vi "Lab Panel V4.86.vi"() -> ()   [LabVIEW 2013] (continued)
                n1197 = case shown="True" w2168 {
                  tunnel: w2173 -> [_ w2177]
                  tunnel: w2167 -> [_ w2180]
                  frame False {
                  }
                  frame True {
                    n1198 = local read "SET LAB01-1"() -> (w2179:T5)
                    n1199 = local read "TDMS LAB01-1"() -> (w2176:refnum<k34>)
                    n1200 = Unbundle(w2177) -> ("CYCLE"=w2181:dbl)  [unwired: 2 out]
                    n1201 = Unbundle(w2179) -> ("T-RISE mins"=w2178:dbl)  [unwired: 4 out]
                    n1202 = Greater Or Equal?(x=w2181, y=w2180) -> (x >= y?=w2182:bool)
                    n1203 = case shown="True" w2182 {
                      tunnel: w2178 -> [w2185 _]
                      tunnel: w2177 -> [w2184 _]
                      tunnel: w2176 -> [w2183 _]
                      frame True {
                        n1204 = stacked-sequence {
                          tunnel: w2185 -> [w2188 _]
                          tunnel: w2184 -> [_ w2193]
                          tunnel: w2183 -> [w2186 _]
                          frame #0 {
                            n1205 = Build Array("T-RISE") -> (w2190:string[])
                            n1206 = Build Array(w2188) -> (w2189:dbl[])
                            n1207 = TDMS Write(0:w2186, 5:"TEST PASS", 7:w2190, 9:w2189) -> (15:w2192:errorcluster)  [unwired: 2 in, 3 out]
                            n1208 = local write "data file error"(w2192) -> ()
                          }
                          frame #1 {
                            n1209 = Bundle(cluster=w2193, "STATUS"="T-RISE PASS") -> (w2195:T4)  [unwired: 2 in]
                            n1210 = local write "RESULT LAB01-1"(TRUE) -> ()
                            n1211 = local write "DISP LAB01-1"(w2195) -> ()
                          }
                        }
                      }
                      frame False {
                      }
                    }
                  }
                }
              }
              frame #1 {
                # "LAB01-2"
                n1212 = Equal?(x=w2198, y=2) -> (x = y?=w2201:bool)
                n1213 = local read "DISP LAB01-2"() -> (w2203:T4)
                n1214 = Unbundle(w2203) -> ("STATUS"=w2204:string)  [unwired: 2 out]
                n1215 = Equal?(x=w2204, y="RUN") -> (x = y?=w2200:bool)
                n1216 = And(x=w2200, y=w2201) -> (x .and. y?=w2199:bool)
                n1217 = case shown="True" w2199 {
                  tunnel: w2203 -> [_ w2207]
                  tunnel: w2197 -> [_ w2210]
                  frame False {
                  }
                  frame True {
                    n1218 = local read "SET LAB01-2"() -> (w2209:T5)
                    n1219 = local read "TDMS LAB01-2"() -> (w2206:refnum<k34>)
                    n1220 = Unbundle(w2207) -> ("CYCLE"=w2211:dbl)  [unwired: 2 out]
                    n1221 = Unbundle(w2209) -> ("T-RISE mins"=w2208:dbl)  [unwired: 4 out]
                    n1222 = Greater Or Equal?(x=w2211, y=w2210) -> (x >= y?=w2212:bool)
                    n1223 = case shown="True" w2212 {
                      tunnel: w2208 -> [w2215 _]
                      tunnel: w2207 -> [w2214 _]
                      tunnel: w2206 -> [w2213 _]
                      frame True {
                        n1224 = stacked-sequence {
                          tunnel: w2215 -> [w2218 _]
                          tunnel: w2214 -> [_ w2223]
                          tunnel: w2213 -> [w2216 _]
                          frame #0 {
                            n1225 = Build Array("T-RISE") -> (w2220:string[])
                            n1226 = Build Array(w2218) -> (w2219:dbl[])
                            n1227 = TDMS Write(0:w2216, 5:"TEST PASS", 7:w2220, 9:w2219) -> (15:w2222:errorcluster)  [unwired: 2 in, 3 out]
                            n1228 = local write "data file error"(w2222) -> ()
                          }
                          frame #1 {
                            n1229 = Bundle(cluster=w2223, "STATUS"="T-RISE PASS") -> (w2225:T4)  [unwired: 2 in]
                            n1230 = local write "RESULT LAB01-2"(TRUE) -> ()
                            n1231 = local write "DISP LAB01-2"(w2225) -> ()
                          }
                        }
                      }
                      frame False {
                      }
                    }
                  }
                }
              }
              frame #2 {
                # "LAB02-1"
                n1232 = Equal?(x=w2228, y=2) -> (x = y?=w2231:bool)
                n1233 = local read "DISP LAB02-1"() -> (w2233:T4)
                n1234 = Unbundle(w2233) -> ("STATUS"=w2234:string)  [unwired: 2 out]
                n1235 = Equal?(x=w2234, y="RUN") -> (x = y?=w2230:bool)
                n1236 = And(x=w2230, y=w2231) -> (x .and. y?=w2229:bool)
                n1237 = case shown="True" w2229 {
                  tunnel: w2233 -> [_ w2237]
                  tunnel: w2227 -> [_ w2240]
                  frame False {
                  }
                  frame True {
                    n1238 = local read "SET LAB02-1"() -> (w2239:T5)
                    n1239 = local read "TDMS LAB02-1"() -> (w2236:refnum<k34>)
                    n1240 = Unbundle(w2237) -> ("CYCLE"=w2241:dbl)  [unwired: 2 out]
                    n1241 = Unbundle(w2239) -> ("T-RISE mins"=w2238:dbl)  [unwired: 4 out]
                    n1242 = Greater Or Equal?(x=w2241, y=w2240) -> (x >= y?=w2242:bool)
                    n1243 = case shown="True" w2242 {
                      tunnel: w2238 -> [w2245 _]
                      tunnel: w2237 -> [w2244 _]
                      tunnel: w2236 -> [w2243 _]
                      frame True {
                        n1244 = stacked-sequence {
                          tunnel: w2245 -> [w2248 _]
                          tunnel: w2244 -> [_ w2253]
                          tunnel: w2243 -> [w2246 _]
                          frame #0 {
                            n1245 = Build Array("T-RISE") -> (w2250:string[])
                            n1246 = Build Array(w2248) -> (w2249:dbl[])
                            n1247 = TDMS Write(0:w2246, 5:"TEST PASS", 7:w2250, 9:w2249) -> (15:w2252:errorcluster)  [unwired: 2 in, 3 out]
                            n1248 = local write "data file error"(w2252) -> ()
                          }
                          frame #1 {
                            n1249 = Bundle(cluster=w2253, "STATUS"="T-RISE PASS") -> (w2255:T4)  [unwired: 2 in]
                            n1250 = local write "RESULT LAB02-1"(TRUE) -> ()
                            n1251 = local write "DISP LAB02-1"(w2255) -> ()
                          }
                        }
                      }
                      frame False {
                      }
                    }
                  }
                }
              }
              frame #3 {
                # "LAB02-2"
                n1252 = Equal?(x=w2258, y=2) -> (x = y?=w2261:bool)
                n1253 = local read "DISP LAB02-2"() -> (w2263:T4)
                n1254 = Unbundle(w2263) -> ("STATUS"=w2264:string)  [unwired: 2 out]
                n1255 = Equal?(x=w2264, y="RUN") -> (x = y?=w2260:bool)
                n1256 = And(x=w2260, y=w2261) -> (x .and. y?=w2259:bool)
                n1257 = case shown="True" w2259 {
                  tunnel: w2263 -> [_ w2267]
                  tunnel: w2257 -> [_ w2270]
                  frame False {
                  }
                  frame True {
                    n1258 = local read "SET LAB02-2"() -> (w2269:T5)
                    n1259 = local read "TDMS LAB02-2"() -> (w2266:refnum<k34>)
                    n1260 = Unbundle(w2267) -> ("CYCLE"=w2271:dbl)  [unwired: 2 out]
                    n1261 = Unbundle(w2269) -> ("T-RISE mins"=w2268:dbl)  [unwired: 4 out]
                    n1262 = Greater Or Equal?(x=w2271, y=w2270) -> (x >= y?=w2272:bool)
                    n1263 = case shown="True" w2272 {
                      tunnel: w2268 -> [w2275 _]
                      tunnel: w2267 -> [w2274 _]
                      tunnel: w2266 -> [w2273 _]
                      frame True {
                        n1264 = stacked-sequence {
                          tunnel: w2275 -> [w2278 _]
                          tunnel: w2274 -> [_ w2283]
                          tunnel: w2273 -> [w2276 _]
                          frame #0 {
                            n1265 = Build Array("T-RISE") -> (w2280:string[])
                            n1266 = Build Array(w2278) -> (w2279:dbl[])
                            n1267 = TDMS Write(0:w2276, 5:"TEST PASS", 7:w2280, 9:w2279) -> (15:w2282:errorcluster)  [unwired: 2 in, 3 out]
                            n1268 = local write "data file error"(w2282) -> ()
                          }
                          frame #1 {
                            n1269 = Bundle(cluster=w2283, "STATUS"="T-RISE PASS") -> (w2285:T4)  [unwired: 2 in]
                            n1270 = local write "RESULT LAB02-2"(TRUE) -> ()
                            n1271 = local write "DISP LAB02-2"(w2285) -> ()
                          }
                        }
                      }
                      frame False {
                      }
                    }
                  }
                }
              }
              frame #4 {
                # "LAB03-1"
                n1272 = Equal?(x=w2288, y=2) -> (x = y?=w2291:bool)
                n1273 = local read "DISP LAB03-1"() -> (w2293:T4)
                n1274 = Unbundle(w2293) -> ("STATUS"=w2294:string)  [unwired: 2 out]
                n1275 = Equal?(x=w2294, y="RUN") -> (x = y?=w2290:bool)
                n1276 = And(x=w2290, y=w2291) -> (x .and. y?=w2289:bool)
                n1277 = case shown="True" w2289 {
                  tunnel: w2293 -> [_ w2297]
                  tunnel: w2287 -> [_ w2300]
                  frame False {
                  }
                  frame True {
                    n1278 = local read "SET LAB03-1"() -> (w2299:T5)
                    n1279 = local read "TDMS LAB03-1"() -> (w2296:refnum<k34>)
                    n1280 = Unbundle(w2297) -> ("CYCLE"=w2301:dbl)  [unwired: 2 out]
                    n1281 = Unbundle(w2299) -> ("T-RISE mins"=w2298:dbl)  [unwired: 4 out]
                    n1282 = Greater Or Equal?(x=w2301, y=w2300) -> (x >= y?=w2302:bool)
                    n1283 = case shown="True" w2302 {
                      tunnel: w2298 -> [w2305 _]
                      tunnel: w2297 -> [w2304 _]
                      tunnel: w2296 -> [w2303 _]
                      frame True {
                        n1284 = stacked-sequence {
                          tunnel: w2305 -> [w2308 _]
                          tunnel: w2304 -> [_ w2313]
                          tunnel: w2303 -> [w2306 _]
                          frame #0 {
                            n1285 = Build Array("T-RISE") -> (w2310:string[])
                            n1286 = Build Array(w2308) -> (w2309:dbl[])
                            n1287 = TDMS Write(0:w2306, 5:"TEST PASS", 7:w2310, 9:w2309) -> (15:w2312:errorcluster)  [unwired: 2 in, 3 out]
                            n1288 = local write "data file error"(w2312) -> ()
                          }
                          frame #1 {
                            n1289 = Bundle(cluster=w2313, "STATUS"="T-RISE PASS") -> (w2315:T4)  [unwired: 2 in]
                            n1290 = local write "RESULT LAB03-1"(TRUE) -> ()
                            n1291 = local write "DISP LAB03-1"(w2315) -> ()
                          }
                        }
                      }
                      frame False {
                      }
                    }
                  }
                }
              }
              frame #5 {
                # "LAB03-2"
                n1292 = Equal?(x=w2318, y=2) -> (x = y?=w2321:bool)
                n1293 = local read "DISP LAB03-2"() -> (w2323:T4)
                n1294 = Unbundle(w2323) -> ("STATUS"=w2324:string)  [unwired: 2 out]
                n1295 = Equal?(x=w2324, y="RUN") -> (x = y?=w2320:bool)
                n1296 = And(x=w2320, y=w2321) -> (x .and. y?=w2319:bool)
                n1297 = case shown="True" w2319 {
                  tunnel: w2323 -> [_ w2327]
                  tunnel: w2317 -> [_ w2330]
                  frame False {
                  }
                  frame True {
                    n1298 = local read "SET LAB03-2"() -> (w2329:T5)
                    n1299 = local read "TDMS LAB03-2"() -> (w2326:refnum<k34>)
                    n1300 = Unbundle(w2327) -> ("CYCLE"=w2331:dbl)  [unwired: 2 out]
                    n1301 = Unbundle(w2329) -> ("T-RISE mins"=w2328:dbl)  [unwired: 4 out]
                    n1302 = Greater Or Equal?(x=w2331, y=w2330) -> (x >= y?=w2332:bool)
                    n1303 = case shown="True" w2332 {
                      tunnel: w2328 -> [w2335 _]
                      tunnel: w2327 -> [w2334 _]
                      tunnel: w2326 -> [w2333 _]
                      frame True {
                        n1304 = stacked-sequence {
                          tunnel: w2335 -> [w2338 _]
                          tunnel: w2334 -> [_ w2343]
                          tunnel: w2333 -> [w2336 _]
                          frame #0 {
                            n1305 = Build Array("T-RISE") -> (w2340:string[])
                            n1306 = Build Array(w2338) -> (w2339:dbl[])
                            n1307 = TDMS Write(0:w2336, 5:"TEST PASS", 7:w2340, 9:w2339) -> (15:w2342:errorcluster)  [unwired: 2 in, 3 out]
                            n1308 = local write "data file error"(w2342) -> ()
                          }
                          frame #1 {
                            n1309 = Bundle(cluster=w2343, "STATUS"="T-RISE PASS") -> (w2345:T4)  [unwired: 2 in]
                            n1310 = local write "RESULT LAB03-2"(TRUE) -> ()
                            n1311 = local write "DISP LAB03-2"(w2345) -> ()
                          }
                        }
                      }
                      frame False {
                      }
                    }
                  }
                }
              }
              frame #6 {
                # "LAB04-1"
                n1312 = Equal?(x=w2348, y=2) -> (x = y?=w2351:bool)
                n1313 = local read "DISP LAB04-1"() -> (w2353:T4)
                n1314 = Unbundle(w2353) -> ("STATUS"=w2354:string)  [unwired: 2 out]
                n1315 = Equal?(x=w2354, y="RUN") -> (x = y?=w2350:bool)
                n1316 = And(x=w2350, y=w2351) -> (x .and. y?=w2349:bool)
                n1317 = case shown="True" w2349 {
                  tunnel: w2353 -> [_ w2357]
                  tunnel: w2347 -> [_ w2360]
                  frame False {
                  }
                  frame True {
                    n1318 = local read "SET LAB04-1"() -> (w2359:T5)
                    n1319 = local read "TDMS LAB04-1"() -> (w2356:refnum<k34>)
                    n1320 = Unbundle(w2357) -> ("CYCLE"=w2361:dbl)  [unwired: 2 out]
                    n1321 = Unbundle(w2359) -> ("T-RISE mins"=w2358:dbl)  [unwired: 4 out]
                    n1322 = Greater Or Equal?(x=w2361, y=w2360) -> (x >= y?=w2362:bool)
                    n1323 = case shown="True" w2362 {
                      tunnel: w2358 -> [w2365 _]
                      tunnel: w2357 -> [w2364 _]
                      tunnel: w2356 -> [w2363 _]
                      frame True {
                        n1324 = stacked-sequence {
                          tunnel: w2365 -> [w2368 _]
                          tunnel: w2364 -> [_ w2373]
                          tunnel: w2363 -> [w2366 _]
                          frame #0 {
                            n1325 = Build Array("T-RISE") -> (w2370:string[])
                            n1326 = Build Array(w2368) -> (w2369:dbl[])
                            n1327 = TDMS Write(0:w2366, 5:"TEST PASS", 7:w2370, 9:w2369) -> (15:w2372:errorcluster)  [unwired: 2 in, 3 out]
                            n1328 = local write "data file error"(w2372) -> ()
                          }
                          frame #1 {
                            n1329 = Bundle(cluster=w2373, "STATUS"="T-RISE PASS") -> (w2375:T4)  [unwired: 2 in]
                            n1330 = local write "RESULT LAB04-1"(TRUE) -> ()
                            n1331 = local write "DISP LAB04-1"(w2375) -> ()
                          }
                        }
                      }
                      frame False {
                      }
                    }
                  }
                }
              }
              frame #7 {
                # "LAB04-2"
                n1332 = Equal?(x=w2378, y=2) -> (x = y?=w2381:bool)
                n1333 = local read "DISP LAB04-2"() -> (w2383:T4)
                n1334 = Unbundle(w2383) -> ("STATUS"=w2384:string)  [unwired: 2 out]
                n1335 = Equal?(x=w2384, y="RUN") -> (x = y?=w2380:bool)
                n1336 = And(x=w2380, y=w2381) -> (x .and. y?=w2379:bool)
                n1337 = case shown="True" w2379 {
                  tunnel: w2383 -> [_ w2387]
                  tunnel: w2377 -> [_ w2390]
                  frame False {
                  }
                  frame True {
                    n1338 = local read "SET LAB04-2"() -> (w2389:T5)
                    n1339 = local read "TDMS LAB04-2"() -> (w2386:refnum<k34>)
                    n1340 = Unbundle(w2387) -> ("CYCLE"=w2391:dbl)  [unwired: 2 out]
                    n1341 = Unbundle(w2389) -> ("T-RISE mins"=w2388:dbl)  [unwired: 4 out]
                    n1342 = Greater Or Equal?(x=w2391, y=w2390) -> (x >= y?=w2392:bool)
                    n1343 = case shown="True" w2392 {
                      tunnel: w2388 -> [w2395 _]
                      tunnel: w2387 -> [w2394 _]
                      tunnel: w2386 -> [w2393 _]
                      frame True {
                        n1344 = stacked-sequence {
                          tunnel: w2395 -> [w2398 _]
                          tunnel: w2394 -> [_ w2403]
                          tunnel: w2393 -> [w2396 _]
                          frame #0 {
                            n1345 = Build Array("T-RISE") -> (w2400:string[])
                            n1346 = Build Array(w2398) -> (w2399:dbl[])
                            n1347 = TDMS Write(0:w2396, 5:"TEST PASS", 7:w2400, 9:w2399) -> (15:w2402:errorcluster)  [unwired: 2 in, 3 out]
                            n1348 = local write "data file error"(w2402) -> ()
                          }
                          frame #1 {
                            n1349 = Bundle(cluster=w2403, "STATUS"="T-RISE PASS") -> (w2405:T4)  [unwired: 2 in]
                            n1350 = local write "RESULT LAB04-2"(TRUE) -> ()
                            n1351 = local write "DISP LAB04-2"(w2405) -> ()
                          }
                        }
                      }
                      frame False {
                      }
                    }
                  }
                }
              }
              frame #8 {
                # "LAB05-1"
                n1352 = Equal?(x=w2408, y=2) -> (x = y?=w2411:bool)
                n1353 = local read "DISP LAB05-1"() -> (w2413:T4)
                n1354 = Unbundle(w2413) -> ("STATUS"=w2414:string)  [unwired: 2 out]
                n1355 = Equal?(x=w2414, y="RUN") -> (x = y?=w2410:bool)
                n1356 = And(x=w2410, y=w2411) -> (x .and. y?=w2409:bool)
                n1357 = case shown="True" w2409 {
                  tunnel: w2413 -> [_ w2417]
                  tunnel: w2407 -> [_ w2420]
                  frame False {
                  }
                  frame True {
                    n1358 = local read "SET LAB05-1"() -> (w2419:T5)
                    n1359 = local read "TDMS LAB05-1"() -> (w2416:refnum<k34>)
                    n1360 = Unbundle(w2417) -> ("CYCLE"=w2421:dbl)  [unwired: 2 out]
                    n1361 = Unbundle(w2419) -> ("T-RISE mins"=w2418:dbl)  [unwired: 4 out]
                    n1362 = Greater Or Equal?(x=w2421, y=w2420) -> (x >= y?=w2422:bool)
                    n1363 = case shown="True" w2422 {
                      tunnel: w2418 -> [w2425 _]
                      tunnel: w2417 -> [w2424 _]
                      tunnel: w2416 -> [w2423 _]
                      frame True {
                        n1364 = stacked-sequence {
                          tunnel: w2425 -> [w2428 _]
                          tunnel: w2424 -> [_ w2433]
                          tunnel: w2423 -> [w2426 _]
                          frame #0 {
                            n1365 = Build Array("T-RISE") -> (w2430:string[])
                            n1366 = Build Array(w2428) -> (w2429:dbl[])
                            n1367 = TDMS Write(0:w2426, 5:"TEST PASS", 7:w2430, 9:w2429) -> (15:w2432:errorcluster)  [unwired: 2 in, 3 out]
                            n1368 = local write "data file error"(w2432) -> ()
                          }
                          frame #1 {
                            n1369 = Bundle(cluster=w2433, "STATUS"="T-RISE PASS") -> (w2435:T4)  [unwired: 2 in]
                            n1370 = local write "RESULT LAB05-1"(TRUE) -> ()
                            n1371 = local write "DISP LAB05-1"(w2435) -> ()
                          }
                        }
                      }
                      frame False {
                      }
                    }
                  }
                }
              }
              frame #9 {
                # "LAB05-2"
                n1372 = Equal?(x=w2438, y=2) -> (x = y?=w2441:bool)
                n1373 = local read "DISP LAB05-2"() -> (w2443:T4)
                n1374 = Unbundle(w2443) -> ("STATUS"=w2444:string)  [unwired: 2 out]
                n1375 = Equal?(x=w2444, y="RUN") -> (x = y?=w2440:bool)
                n1376 = And(x=w2440, y=w2441) -> (x .and. y?=w2439:bool)
                n1377 = case shown="True" w2439 {
                  tunnel: w2443 -> [_ w2447]
                  tunnel: w2437 -> [_ w2450]
                  frame False {
                  }
                  frame True {
                    n1378 = local read "SET LAB05-2"() -> (w2449:T5)
                    n1379 = local read "TDMS LAB05-2"() -> (w2446:refnum<k34>)
                    n1380 = Unbundle(w2447) -> ("CYCLE"=w2451:dbl)  [unwired: 2 out]
                    n1381 = Unbundle(w2449) -> ("T-RISE mins"=w2448:dbl)  [unwired: 4 out]
                    n1382 = Greater Or Equal?(x=w2451, y=w2450) -> (x >= y?=w2452:bool)
                    n1383 = case shown="True" w2452 {
                      tunnel: w2448 -> [w2455 _]
                      tunnel: w2447 -> [w2454 _]
                      tunnel: w2446 -> [w2453 _]
                      frame True {
                        n1384 = stacked-sequence {
                          tunnel: w2455 -> [w2458 _]
                          tunnel: w2454 -> [_ w2463]
                          tunnel: w2453 -> [w2456 _]
                          frame #0 {
                            n1385 = Build Array("T-RISE") -> (w2460:string[])
                            n1386 = Build Array(w2458) -> (w2459:dbl[])
                            n1387 = TDMS Write(0:w2456, 5:"TEST PASS", 7:w2460, 9:w2459) -> (15:w2462:errorcluster)  [unwired: 2 in, 3 out]
                            n1388 = local write "data file error"(w2462) -> ()
                          }
                          frame #1 {
                            n1389 = Bundle(cluster=w2463, "STATUS"="T-RISE PASS") -> (w2465:T4)  [unwired: 2 in]
                            n1390 = local write "RESULT LAB05-2"(TRUE) -> ()
                            n1391 = local write "DISP LAB05-2"(w2465) -> ()
                          }
                        }
                      }
                      frame False {
                      }
                    }
                  }
                }
              }
            }
          }
          frame #6 {
            # "end test & close test files"
            n1392 = local read "MAIL SETTINGS"() -> (w2471:T6)
            n1393 = Unbundle(w2471) -> ("OUT SERVER ADDRESS"=w2470:string, "FROM ACCOUNT"=w2469:string)  [unwired: 5 out]
            n1394 = stacked-sequence {
              tunnel: w2481 -> [_ _ _ _ _ _ _ _ _ _]
              tunnel: w2482 -> [_ _ _ _ _ _ _ _ _ _]
              tunnel: w2480 -> [_ _ _ _ _ _ _ _ _ _]
              tunnel: w2479 -> [_ _ _ _ _ _ _ _ _ _]
              tunnel: w2478 -> [_ _ _ _ _ _ _ _ _ _]
              tunnel: w2477 -> [_ _ _ _ _ _ _ _ _ _]
              tunnel: w2476 -> [_ _ _ _ _ _ _ _ _ _]
              tunnel: w2475 -> [_ _ _ _ _ _ _ _ _ _]
              tunnel: w2474 -> [_ _ _ _ _ _ _ _ _ _]
              tunnel: w2473 -> [_ _ _ _ _ _ _ _ _ _]
              tunnel: w2470 -> [w2486 w2538 w2586 w2633 w2680 w2727 w2774 w2821 w2868 w2915]
              tunnel: w2469 -> [w2485 w2537 w2585 w2632 w2679 w2726 w2773 w2820 w2867 w2914]
              tunnel: "Mail Test File To:" -> [w2484 w2536 w2584 w2631 w2678 w2725 w2772 w2819 w2866 w2913]
              tunnel: "Mail Test Fail" -> [w2483 w2535 w2583 w2630 w2677 w2724 w2771 w2818 w2865 w2912]
              frame #0 {
                # "LAB01-1"
                n1395 = local read "DISP LAB01-1"() -> (w2490:T4)
                n1396 = local read "run lab01-1"() -> (w2487:bool)
                n1397 = local read "TDMS LAB01-1"() -> (w2488:refnum<k34>)
                n1398 = Unbundle(w2490) -> ("CYCLE"=w2491:dbl, "STATUS"=w2489:string)  [unwired: 1 out]
                n1399 = case shown="True" w2487 {
                  tunnel: w2491 -> [_ w2497]
                  tunnel: w2490 -> [_ w2499]
                  tunnel: w2489 -> [_ w2496]
                  tunnel: w2488 -> [_ w2498]
                  tunnel: w2486 -> [_ w2495]
                  tunnel: w2485 -> [_ w2494]
                  tunnel: w2484 -> [_ w2493]
                  tunnel: w2483 -> [_ w2492]
                  frame False {
                  }
                  frame True {
                    n1400 = Not Equal?(x=w2496, y="RUN") -> (x != y?=w2500:bool)
                    n1401 = Greater?(x=w2497, y=2.0) -> (0:w2502:bool)
                    n1402 = And(x=w2502, y=w2500) -> (x .and. y?=w2501:bool)
                    n1403 = case shown="True" w2501 {
                      tunnel: w2499 -> [_ w2512]
                      tunnel: w2498 -> [_ w2511]
                      tunnel: w2497 -> [_ w2510]
                      tunnel: w2496 -> [_ w2509]
                      tunnel: w2495 -> [_ w2508]
                      tunnel: w2494 -> [_ w2507]
                      tunnel: w2493 -> [_ w2506]
                      tunnel: w2492 -> [_ w2505]
                      frame False {
                      }
                      frame True {
                        n1404 = stacked-sequence {
                          tunnel: w2512 -> [w2516 _ _]
                          tunnel: w2511 -> [_ w2518 _]
                          tunnel: w2510 -> [_ _ _]
                          tunnel: w2509 -> [_ _ w2524]
                          tunnel: w2508 -> [_ _ w2523]
                          tunnel: w2507 -> [_ _ w2522]
                          tunnel: w2506 -> [_ _ w2521]
                          tunnel: w2505 -> [_ _ w2520]
                          frame #0 {
                            w2513 = FALSE
                            n1405 = local write "mail control"("END") -> ()
                            n1406 = Bundle(cluster=w2516) -> (w2515:T4)  [unwired: 3 in]
                            n1407 = local write "DISP LAB01-1"(w2515) -> ()
                            n1408 = local write "O/I  LAB01-1"(w2513) -> ()
                            n1409 = local write "run lab01-1"(w2513) -> ()
                            n1410 = local write "RUN LAB01-1"(w2513) -> ()
                          }
                          frame #1 {
                            n1411 = TDMS Close(11:w2518) -> (0:w2517:errorcluster)  [unwired: 1 in, 1 out]
                            n1412 = local write "data file error"(w2517) -> ()
                          }
                          frame #2 {
                            n1413 = stacked-sequence {
                              tunnel: "LAB01-1" -> [w2526 w2528 _]
                              tunnel: w2524 -> [_ w2534 _]
                              tunnel: w2523 -> [_ w2533 _]
                              tunnel: w2522 -> [_ w2532 _]
                              tunnel: w2521 -> [_ w2531 _]
                              tunnel: w2520 -> [_ w2530 _]
                              frame #0 {
                                n1414 = call "sub vi - defrag tdms v1.vi"("panel id"=w2526) -> ("error out"=w2525:errorcluster)  [unwired: 10 in]
                                n1415 = local write "data file error"(w2525) -> ()
                              }
                              frame #1 {
                                n1416 = Bundle("STATUS"=w2534, "OUT SERVER ADDRESS"=w2533, "FROM ACCOUNT"=w2532, "Mail Test File To:"=w2531, "Mail Test Fail"=w2530) -> (w2527:T23)  [unwired: 1 in]
                                n1417 = call "Save data file to network drive v3.vi"("Input Cluster"=w2527, "panel id"=w2528) -> ("network file save error"=w2529:errorcluster)  [unwired: 8 in, 1 out]
                                n1418 = local write "data file error"(w2529) -> ()
                              }
                              frame #2 {
                              }
                            }
                          }
                        }
                      }
                    }
                  }
                }
              }
              frame #1 {
                # "LAB01-2"
                n1419 = local read "run lab01-2"() -> (w2539:bool)
                n1420 = case shown="True" w2539 {
                  tunnel: w2538 -> [_ w2543]
                  tunnel: w2537 -> [_ w2542]
                  tunnel: w2536 -> [_ w2541]
                  tunnel: w2535 -> [_ w2540]
                  frame False {
                  }
                  frame True {
                    n1421 = local read "DISP LAB01-2"() -> (w2551:T4)
                    n1422 = local read "TDMS LAB01-2"() -> (w2550:refnum<k34>)
                    n1423 = Unbundle(w2551) -> ("CYCLE"=w2545:dbl, "STATUS"=w2544:string)  [unwired: 1 out]
                    n1424 = Not Equal?(x=w2544, y="RUN") -> (x != y?=w2547:bool)
                    n1425 = Greater?(x=w2545, y=2.0) -> (0:w2548:bool)
                    n1426 = And(x=w2548, y=w2547) -> (x .and. y?=w2546:bool)
                    n1427 = case shown="True" w2546 {
                      tunnel: w2551 -> [_ w2560]
                      tunnel: w2550 -> [_ w2559]
                      tunnel: w2545 -> [_ w2558]
                      tunnel: w2544 -> [_ w2557]
                      tunnel: w2543 -> [_ w2556]
                      tunnel: w2542 -> [_ w2555]
                      tunnel: w2541 -> [_ w2554]
                      tunnel: w2540 -> [_ w2553]
                      frame False {
                      }
                      frame True {
                        n1428 = stacked-sequence {
                          tunnel: w2560 -> [w2563 _ _]
                          tunnel: w2559 -> [_ w2565 _]
                          tunnel: w2558 -> [_ _ _]
                          tunnel: w2557 -> [_ _ w2571]
                          tunnel: w2556 -> [_ _ w2570]
                          tunnel: w2555 -> [_ _ w2569]
                          tunnel: w2554 -> [_ _ w2568]
                          tunnel: w2553 -> [_ _ w2567]
                          frame #0 {
                            w2561 = FALSE
                            n1429 = local write "mail control"("END") -> ()
                            n1430 = Bundle(cluster=w2563) -> (w2564:T4)  [unwired: 3 in]
                            n1431 = local write "RUN LAB01-2"(w2561) -> ()
                            n1432 = local write "run lab01-2"(w2561) -> ()
                            n1433 = local write "O/I  LAB01-2"(w2561) -> ()
                            n1434 = local write "DISP LAB01-2"(w2564) -> ()
                          }
                          frame #1 {
                            n1435 = TDMS Close(11:w2565) -> (0:w2566:errorcluster)  [unwired: 1 in, 1 out]
                            n1436 = local write "data file error"(w2566) -> ()
                          }
                          frame #2 {
                            n1437 = stacked-sequence {
                              tunnel: "LAB01-2" -> [w2574 w2575]
                              tunnel: w2571 -> [_ w2580]
                              tunnel: w2570 -> [_ w2579]
                              tunnel: w2569 -> [_ w2578]
                              tunnel: w2568 -> [_ w2577]
                              tunnel: w2567 -> [_ w2576]
                              frame #0 {
                                n1438 = call "sub vi - defrag tdms v1.vi"("panel id"=w2574) -> ("error out"=w2573:errorcluster)  [unwired: 10 in]
                                n1439 = local write "data file error"(w2573) -> ()
                              }
                              frame #1 {
                                n1440 = Bundle("STATUS"=w2580, "OUT SERVER ADDRESS"=w2579, "FROM ACCOUNT"=w2578, "Mail Test File To:"=w2577, "Mail Test Fail"=w2576) -> (w2582:T23)  [unwired: 1 in]
                                n1441 = call "Save data file to network drive v3.vi"("Input Cluster"=w2582, "panel id"=w2575) -> ("network file save error"=w2581:errorcluster)  [unwired: 8 in, 1 out]
                                n1442 = local write "data file error"(w2581) -> ()
                              }
                            }
                          }
                        }
                      }
                    }
                  }
                }
              }
              frame #2 {
                # "LAB02-1"
                n1443 = local read "run lab02-1"() -> (w2587:bool)
                n1444 = case shown="True" w2587 {
                  tunnel: w2586 -> [_ w2591]
                  tunnel: w2585 -> [_ w2590]
                  tunnel: w2584 -> [_ w2589]
                  tunnel: w2583 -> [_ w2588]
                  frame False {
                  }
                  frame True {
                    n1445 = local read "DISP LAB02-1"() -> (w2599:T4)
                    n1446 = Unbundle(w2599) -> ("CYCLE"=w2595:dbl, "STATUS"=w2592:string)  [unwired: 1 out]
                    n1447 = local read "TDMS LAB02-1"() -> (w2598:refnum<k34>)
                    n1448 = Not Equal?(x=w2592, y="RUN") -> (x != y?=w2594:bool)
                    n1449 = Greater?(x=w2595, y=2.0) -> (0:w2596:bool)
                    n1450 = And(x=w2596, y=w2594) -> (x .and. y?=w2593:bool)
                    n1451 = case shown="True" w2593 {
                      tunnel: w2599 -> [_ w2607]
                      tunnel: w2598 -> [_ w2606]
                      tunnel: w2592 -> [_ w2605]
                      tunnel: w2591 -> [_ w2604]
                      tunnel: w2590 -> [_ w2603]
                      tunnel: w2589 -> [_ w2602]
                      tunnel: w2588 -> [_ w2601]
                      frame False {
                      }
                      frame True {
                        n1452 = stacked-sequence {
                          tunnel: w2607 -> [w2610 _ _]
                          tunnel: w2606 -> [_ w2612 _]
                          tunnel: w2605 -> [_ _ w2618]
                          tunnel: w2604 -> [_ _ w2617]
                          tunnel: w2603 -> [_ _ w2616]
                          tunnel: w2602 -> [_ _ w2615]
                          tunnel: w2601 -> [_ _ w2614]
                          frame #0 {
                            w2608 = FALSE
                            n1453 = local write "mail control"("END") -> ()
                            n1454 = Bundle(cluster=w2610) -> (w2611:T4)  [unwired: 3 in]
                            n1455 = local write "O/I  LAB02-1"(w2608) -> ()
                            n1456 = local write "RUN LAB02-1"(w2608) -> ()
                            n1457 = local write "run lab02-1"(w2608) -> ()
                            n1458 = local write "DISP LAB02-1"(w2611) -> ()
                          }
                          frame #1 {
                            n1459 = TDMS Close(11:w2612) -> (0:w2613:errorcluster)  [unwired: 1 in, 1 out]
                            n1460 = local write "data file error"(w2613) -> ()
                          }
                          frame #2 {
                            n1461 = stacked-sequence {
                              tunnel: "LAB02-1" -> [w2621 w2628]
                              tunnel: w2618 -> [_ w2626]
                              tunnel: w2617 -> [_ w2625]
                              tunnel: w2616 -> [_ w2624]
                              tunnel: w2615 -> [_ w2623]
                              tunnel: w2614 -> [_ w2622]
                              frame #0 {
                                n1462 = call "sub vi - defrag tdms v1.vi"("panel id"=w2621) -> ("error out"=w2620:errorcluster)  [unwired: 10 in]
                                n1463 = local write "data file error"(w2620) -> ()
                              }
                              frame #1 {
                                n1464 = Bundle("STATUS"=w2626, "OUT SERVER ADDRESS"=w2625, "FROM ACCOUNT"=w2624, "Mail Test File To:"=w2623, "Mail Test Fail"=w2622) -> (w2627:T23)  [unwired: 1 in]
                                n1465 = call "Save data file to network drive v3.vi"("Input Cluster"=w2627, "panel id"=w2628) -> ("network file save error"=w2629:errorcluster)  [unwired: 8 in, 1 out]
                                n1466 = local write "data file error"(w2629) -> ()
                              }
                            }
                          }
                        }
                      }
                    }
                  }
                }
              }
              frame #3 {
                # "LAB02-2"
                n1467 = local read "run lab02-2"() -> (w2634:bool)
                n1468 = case shown="True" w2634 {
                  tunnel: w2633 -> [_ w2638]
                  tunnel: w2632 -> [_ w2637]
                  tunnel: w2631 -> [_ w2636]
                  tunnel: w2630 -> [_ w2635]
                  frame False {
                  }
                  frame True {
                    n1469 = local read "DISP LAB02-2"() -> (w2646:T4)
                    n1470 = local read "TDMS LAB02-2"() -> (w2645:refnum<k34>)
                    n1471 = Unbundle(w2646) -> ("CYCLE"=w2642:dbl, "STATUS"=w2639:string)  [unwired: 1 out]
                    n1472 = Not Equal?(x=w2639, y="RUN") -> (x != y?=w2641:bool)
                    n1473 = Greater?(x=w2642, y=2.0) -> (0:w2643:bool)
                    n1474 = And(x=w2643, y=w2641) -> (x .and. y?=w2640:bool)
                    n1475 = case shown="True" w2640 {
                      tunnel: w2646 -> [_ w2654]
                      tunnel: w2645 -> [_ w2653]
                      tunnel: w2639 -> [_ w2652]
                      tunnel: w2638 -> [_ w2651]
                      tunnel: w2637 -> [_ w2650]
                      tunnel: w2636 -> [_ w2649]
                      tunnel: w2635 -> [_ w2648]
                      frame False {
                      }
                      frame True {
                        n1476 = stacked-sequence {
                          tunnel: w2654 -> [w2657 _ _]
                          tunnel: w2653 -> [_ w2659 _]
                          tunnel: w2652 -> [_ _ w2665]
                          tunnel: w2651 -> [_ _ w2664]
                          tunnel: w2650 -> [_ _ w2663]
                          tunnel: w2649 -> [_ _ w2662]
                          tunnel: w2648 -> [_ _ w2661]
                          frame #0 {
                            w2655 = FALSE
                            n1477 = local write "mail control"("END") -> ()
                            n1478 = Bundle(cluster=w2657) -> (w2658:T4)  [unwired: 3 in]
                            n1479 = local write "O/I  LAB02-2"(w2655) -> ()
                            n1480 = local write "run lab02-2"(w2655) -> ()
                            n1481 = local write "RUN LAB02-2"(w2655) -> ()
                            n1482 = local write "DISP LAB02-2"(w2658) -> ()
                          }
                          frame #1 {
                            n1483 = TDMS Close(11:w2659) -> (0:w2660:errorcluster)  [unwired: 1 in, 1 out]
                            n1484 = local write "data file error"(w2660) -> ()
                          }
                          frame #2 {
                            n1485 = stacked-sequence {
                              tunnel: "LAB02-2" -> [w2668 w2674]
                              tunnel: w2665 -> [_ w2673]
                              tunnel: w2664 -> [_ w2672]
                              tunnel: w2663 -> [_ w2671]
                              tunnel: w2662 -> [_ w2670]
                              tunnel: w2661 -> [_ w2669]
                              frame #0 {
                                n1486 = call "sub vi - defrag tdms v1.vi"("panel id"=w2668) -> ("error out"=w2667:errorcluster)  [unwired: 10 in]
                                n1487 = local write "data file error"(w2667) -> ()
                              }
                              frame #1 {
                                n1488 = Bundle("STATUS"=w2673, "OUT SERVER ADDRESS"=w2672, "FROM ACCOUNT"=w2671, "Mail Test File To:"=w2670, "Mail Test Fail"=w2669) -> (w2676:T23)  [unwired: 1 in]
                                n1489 = call "Save data file to network drive v3.vi"("Input Cluster"=w2676, "panel id"=w2674) -> ("network file save error"=w2675:errorcluster)  [unwired: 8 in, 1 out]
                                n1490 = local write "data file error"(w2675) -> ()
                              }
                            }
                          }
                        }
                      }
                    }
                  }
                }
              }
              frame #4 {
                # "LAB03-1"
                n1491 = local read "run lab03-1"() -> (w2681:bool)
                n1492 = case shown="True" w2681 {
                  tunnel: w2680 -> [_ w2685]
                  tunnel: w2679 -> [_ w2684]
                  tunnel: w2678 -> [_ w2683]
                  tunnel: w2677 -> [_ w2682]
                  frame False {
                  }
                  frame True {
                    n1493 = local read "DISP LAB03-1"() -> (w2693:T4)
                    n1494 = local read "TDMS LAB03-1"() -> (w2692:refnum<k34>)
                    n1495 = Unbundle(w2693) -> ("CYCLE"=w2689:dbl, "STATUS"=w2686:string)  [unwired: 1 out]
                    n1496 = Not Equal?(x=w2686, y="RUN") -> (x != y?=w2688:bool)
                    n1497 = Greater?(x=w2689, y=2.0) -> (0:w2690:bool)
                    n1498 = And(x=w2690, y=w2688) -> (x .and. y?=w2687:bool)
                    n1499 = case shown="True" w2687 {
                      tunnel: w2693 -> [_ w2701]
                      tunnel: w2692 -> [_ w2700]
                      tunnel: w2686 -> [_ w2699]
                      tunnel: w2685 -> [_ w2698]
                      tunnel: w2684 -> [_ w2697]
                      tunnel: w2683 -> [_ w2696]
                      tunnel: w2682 -> [_ w2695]
                      frame False {
                      }
                      frame True {
                        n1500 = stacked-sequence {
                          tunnel: w2701 -> [w2704 _ _]
                          tunnel: w2700 -> [_ w2706 _]
                          tunnel: w2699 -> [_ _ w2712]
                          tunnel: w2698 -> [_ _ w2711]
                          tunnel: w2697 -> [_ _ w2710]
                          tunnel: w2696 -> [_ _ w2709]
                          tunnel: w2695 -> [_ _ w2708]
                          frame #0 {
                            w2702 = FALSE
                            n1501 = local write "mail control"("END") -> ()
                            n1502 = Bundle(cluster=w2704) -> (w2705:T4)  [unwired: 3 in]
                            n1503 = local write "O/I  LAB03-1"(w2702) -> ()
                            n1504 = local write "run lab03-1"(w2702) -> ()
                            n1505 = local write "RUN LAB03-1"(w2702) -> ()
                            n1506 = local write "DISP LAB03-1"(w2705) -> ()
                          }
                          frame #1 {
                            n1507 = TDMS Close(11:w2706) -> (0:w2707:errorcluster)  [unwired: 1 in, 1 out]
                            n1508 = local write "data file error"(w2707) -> ()
                          }
                          frame #2 {
                            n1509 = stacked-sequence {
                              tunnel: "LAB03-1" -> [w2715 w2721]
                              tunnel: w2712 -> [_ w2720]
                              tunnel: w2711 -> [_ w2719]
                              tunnel: w2710 -> [_ w2718]
                              tunnel: w2709 -> [_ w2717]
                              tunnel: w2708 -> [_ w2716]
                              frame #0 {
                                n1510 = call "sub vi - defrag tdms v1.vi"("panel id"=w2715) -> ("error out"=w2714:errorcluster)  [unwired: 10 in]
                                n1511 = local write "data file error"(w2714) -> ()
                              }
                              frame #1 {
                                n1512 = Bundle("STATUS"=w2720, "OUT SERVER ADDRESS"=w2719, "FROM ACCOUNT"=w2718, "Mail Test File To:"=w2717, "Mail Test Fail"=w2716) -> (w2723:T23)  [unwired: 1 in]
                                n1513 = call "Save data file to network drive v3.vi"("Input Cluster"=w2723, "panel id"=w2721) -> ("network file save error"=w2722:errorcluster)  [unwired: 8 in, 1 out]
                                n1514 = local write "data file error"(w2722) -> ()
                              }
                            }
                          }
                        }
                      }
                    }
                  }
                }
              }
              frame #5 {
                # "LAB03-2"
                n1515 = local read "run lab03-2"() -> (w2728:bool)
                n1516 = case shown="True" w2728 {
                  tunnel: w2727 -> [_ w2732]
                  tunnel: w2726 -> [_ w2731]
                  tunnel: w2725 -> [_ w2730]
                  tunnel: w2724 -> [_ w2729]
                  frame False {
                  }
                  frame True {
                    n1517 = local read "DISP LAB03-2"() -> (w2740:T4)
                    n1518 = Unbundle(w2740) -> ("CYCLE"=w2736:dbl, "STATUS"=w2733:string)  [unwired: 1 out]
                    n1519 = local read "TDMS LAB03-2"() -> (w2739:refnum<k34>)
                    n1520 = Not Equal?(x=w2733, y="RUN") -> (x != y?=w2735:bool)
                    n1521 = Greater?(x=w2736, y=2.0) -> (0:w2737:bool)
                    n1522 = And(x=w2737, y=w2735) -> (x .and. y?=w2734:bool)
                    n1523 = case shown="True" w2734 {
                      tunnel: w2740 -> [_ w2748]
                      tunnel: w2739 -> [_ w2747]
                      tunnel: w2733 -> [_ w2746]
                      tunnel: w2732 -> [_ w2745]
                      tunnel: w2731 -> [_ w2744]
                      tunnel: w2730 -> [_ w2743]
                      tunnel: w2729 -> [_ w2742]
                      frame False {
                      }
                      frame True {
                        n1524 = stacked-sequence {
                          tunnel: w2748 -> [w2751 _ _]
                          tunnel: w2747 -> [_ w2753 _]
                          tunnel: w2746 -> [_ _ w2759]
                          tunnel: w2745 -> [_ _ w2758]
                          tunnel: w2744 -> [_ _ w2757]
                          tunnel: w2743 -> [_ _ w2756]
                          tunnel: w2742 -> [_ _ w2755]
                          frame #0 {
                            w2749 = FALSE
                            n1525 = local write "mail control"("END") -> ()
                            n1526 = Bundle(cluster=w2751) -> (w2752:T4)  [unwired: 3 in]
                            n1527 = local write "RUN LAB03-2"(w2749) -> ()
                            n1528 = local write "O/I  LAB03-2"(w2749) -> ()
